vi "LaserCal-mW to V.vi"(0 "I-O":T1, 5 "Power (mW)":dbl, 7 "Pulse width (us)":dbl, 9 "Pulse rate (Hz)":dbl, 11 "error in (no error)":errorcluster) -> (4 "Volts":dbl, 8 "Max (mW)":dbl, 15 "error out":errorcluster)   [LabVIEW 2020]
uses:
  epl-vi-lib/Utility VIs/Math VIs/interp1.vi
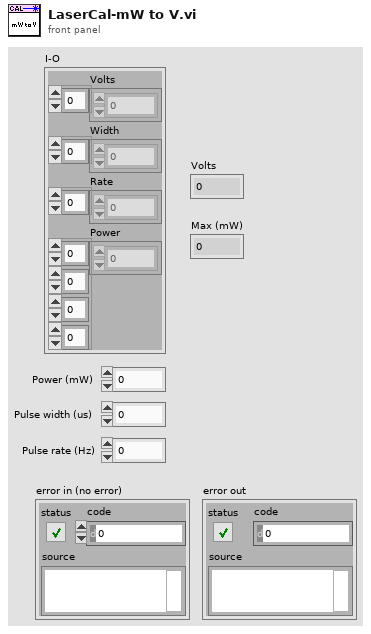
[diagram p1: front panel]
types:
  T1 = cluster{"Volts":dbl[], "Width":dbl[], "Rate":dbl[], "Power":dbl[][][][]}
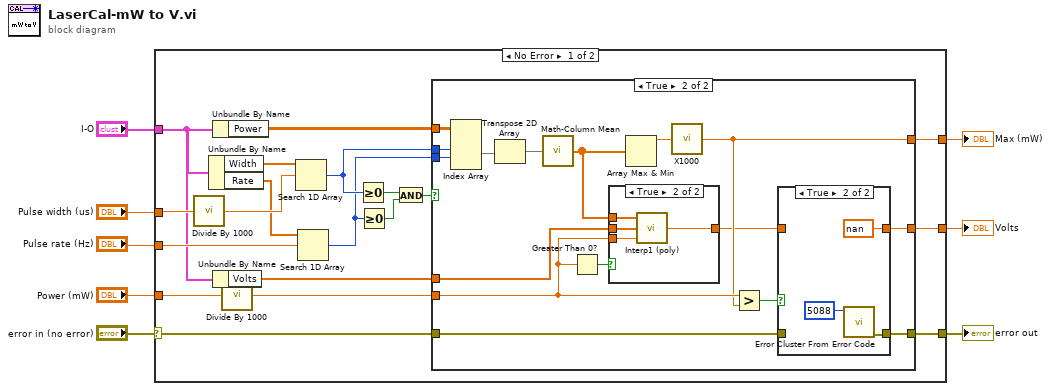
[diagram p0: block diagram]
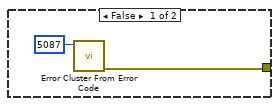
[diagram p2: hidden frame]
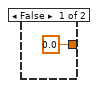
[diagram p4: hidden frame]
diagram:
  n1 = case shown="No Error" "error in (no error)" {
    selector: "error in (no error)" -> [w10 w56]
    tunnel: [w9 w56] -> w6
    tunnel: "Pulse width (us)" -> [w27 _]
    tunnel: "Pulse rate (Hz)" -> [w23 _]
    tunnel: [w18 _] -> w2
    tunnel: "I-O" -> [w21 _]
    tunnel: "Power (mW)" -> [w19 _]
    tunnel: [w16 _] -> w1
    frame No Error {
      n2 = call "Divide By 1000.vi"("X"=w27) -> ("X/1000"=w25:dbl)
      n3 = Unbundle By Name(w21) -> ("Width"=w26:dbl[], "Rate"=w24:dbl[])
      n4 = Unbundle By Name(w21) -> ("Power"=w22:dbl[][][][])
      n5 = Unbundle By Name(w21) -> ("Volts"=w20:dbl[])
      n6 = call "Divide By 1000.vi"("X"=w19) -> ("X/1000"=w17:dbl)
      n7 = Search 1D Array(1D array=w26, element=w25) -> (index of element=w15:i32)  [unwired: 1 in]
      n8 = Search 1D Array(1D array=w24, element=w23) -> (index of element=w14:i32)  [unwired: 1 in]
      n9 = Greater Or Equal To 0?(x=w15) -> (x >= 0?=w13:bool)
      n10 = Greater Or Equal To 0?(x=w14) -> (x >= 0?=w12:bool)
      n11 = And(x=w13, y=w12) -> (x .and. y?=w11:bool)
      n12 = case shown="True" w11 {
        tunnel: w22 -> [_ w45]
        tunnel: w20 -> [_ w42]
        tunnel: [_ w32] -> w18
        tunnel: w17 -> [_ w36]
        tunnel: [_ w35] -> w16
        tunnel: w15 -> [_ w39]
        tunnel: w14 -> [_ w38]
        tunnel: w10 -> [_ w30]
        tunnel: [w29 w31] -> w9
        frame False {
          n13 = call <vilib>:"Error Cluster From Error Code.vi"("error code (0)"=5087) -> ("error out"=w29:errorcluster)  [unwired: 8 in]
        }
        frame True {
          n14 = Index Array(array=w45, index (dim 1)=w39, index (dim 2)=w38) -> (element=w44:dbl[][])  [unwired: 2 in]
          n15 = Transpose 2D Array(2D array=w44) -> (transposed array=w43:dbl[][])
          n16 = call "Math-Column Mean.vi"("2D Array"=w43) -> ("Column means"=w41:dbl[])
          n17 = Greater Than 0?(x=w36) -> (x > 0?=w37:bool)
          n18 = case shown="True" w37 {
            tunnel: w42 -> [_ w55]
            tunnel: [0.0 ("V") w54] -> w33
            tunnel: w36 -> [_ w53]
            tunnel: w41 -> [_ w52]
            frame False {
            }
            frame True {
              n19 = call-poly "Interp1 (poly).vi"("X"=w52, "Y"=w55, "U"=w53) -> ("V"=w54:dbl)  [unwired: 2 in]
            }
          }
          n20 = Array Max & Min(array=w41) -> (max value=w40:dbl)  [unwired: 3 out]
          n21 = call "X1000.vi"("X"=w40) -> ("X/1000"=w35:dbl)
          n22 = Greater?(x=w36, y=w35) -> (0:w34:bool)
          n23 = case shown="True" w34 {
            tunnel: w33 -> [w47 _]
            tunnel: [w47 nan ("V")] -> w32
            tunnel: [w46 w49] -> w31
            tunnel: w30 -> [w46 _]
            frame False {
            }
            frame True {
              n24 = call <vilib>:"Error Cluster From Error Code.vi"("error code (0)"=5088) -> ("error out"=w49:errorcluster)  [unwired: 8 in]
            }
          }
        }
      }
    }
    frame Error {
    }
  }
  "Volts" <- w2
  "error out" <- w6
  "Max (mW)" <- w1
